vi "CreateControlConstructor.vi"(7 "Control in":refnum<class "Control.lvclass">, 8 "error in":errorcluster, 11 "PythonConverter_GUI in":refnum<class "PythonConverter_GUI.lvclass">) -> (0 "error out":errorcluster, 3 "PythonConverter_GUI out":refnum<class "PythonConverter_GUI.lvclass">, 4 "control name":string, 5 "Control out":refnum<class "Control.lvclass">, 6 "control":string)   [LabVIEW 2014, in "PythonConverter_GUI.lvclass"]
uses:
  PythonConverter_GUI.lvclass
  VI Interpreter/Classes/Control/Control.lvclass
  Parsing/Python Functions.lvlib
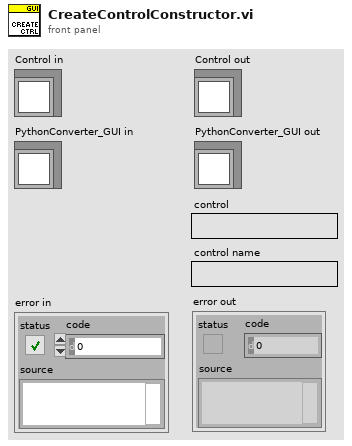
[diagram p1: front panel]
types:
  T1 = typedef "PythonConverter_GUI.lvclass/FPOwnerClassTD.ctl" = enum16{"Panel", "Array", "Cluster", "Tab control"}
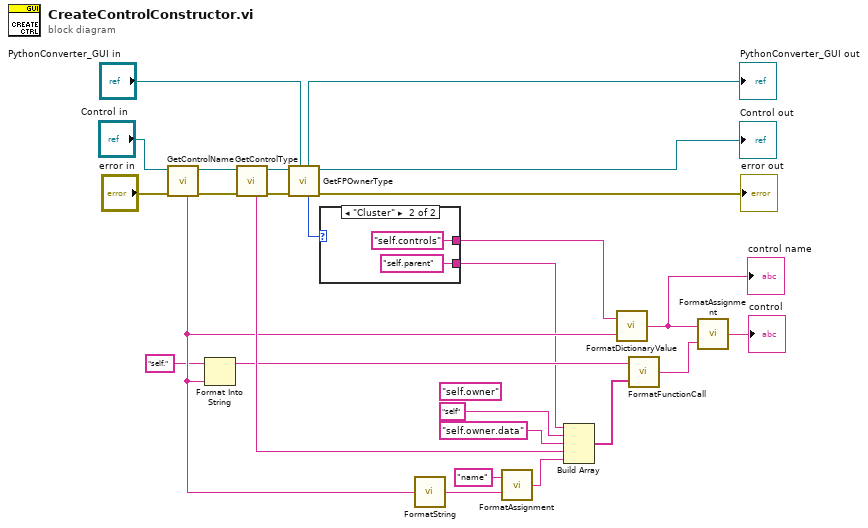
[diagram p0: block diagram]
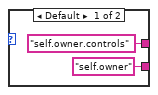
[diagram p2: hidden frame]
diagram:
  (unwired) "self.owner" ("String")
  n1 = call "GetControlName.vi"("error in"="error in", "Control in"="Control in") -> ("error out"=w19:errorcluster, "Control out"=w20:refnum<class "Control.lvclass">, "name"=w12:string)  [unwired: 5 in]
  n2 = Format Into String(initial string="self.", w12) -> (resulting string=w13:string)  [unwired: 2 in, 1 out]
  n3 = call "GetControlType.vi"("error in"=w19, "Control in"=w20) -> ("error out"=w8:errorcluster, "Control out"=w9:refnum<class "Control.lvclass">, "type string"=w23:string)  [unwired: 7 in]
  n4 = call "GetFPOwnerType.vi"("PythonConverter_GUI in"="PythonConverter_GUI in", "error in"=w8, "Object in"=w9) -> ("error out"=→"error out":errorcluster, "Object out"=→"Control out":refnum<class "Control.lvclass">, "owner"=w3:T1, "PythonConverter_GUI out"=→"PythonConverter_GUI out":refnum<class "PythonConverter_GUI.lvclass">)  [unwired: 5 in]
  n5 = case shown="\"Cluster\"" w3 {
    tunnel: ["self.owner.controls" ("dictionary") "self.controls" ("dictionary")] -> w2
    tunnel: ["self.owner" ("String") "self.parent" ("String")] -> w1
    frame Default {
    }
    frame "Cluster" {
    }
  }
  n6 = call "FormatString.vi"("value"=w12) -> ("python object"=w18:string)
  n7 = call "FormatAssignment.vi"("value"=w18, "name"="name") -> ("python assignment"=w21:string)
  n8 = Build Array(w1, "self" ("String"), "self.owner.data" ("String"), w23, w21) -> (w24:string[])
  n9 = call "FormatDictionaryValue.vi"("key"=w12, "dictionary"=w2) -> ("python object"=w14:string)
  "control name" <- w14
  n10 = call "FormatFunctionCall.vi"("parameters"=w24, "function"=w13) -> ("python object"=w26:string)
  n11 = call "FormatAssignment.vi"("value"=w26, "name"=w14) -> ("python assignment"=→"control":string)
